vi "listbox_redrow.vi"() -> ()   [LabVIEW 2021]
panel:
  in  "Red Rows Index":i32[](array[numeric])=[1, 3, 7]
  out "Multicolumn Listbox":i32[](listbox)
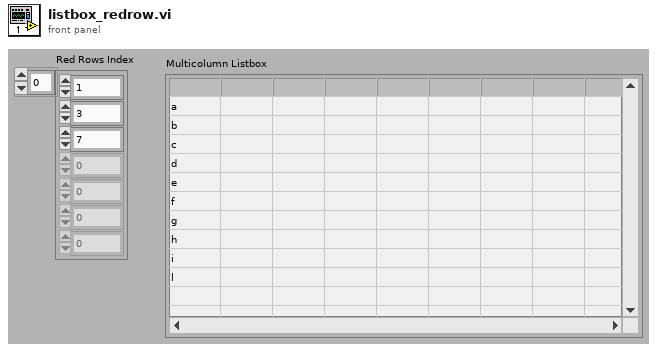
[diagram p1: front panel]
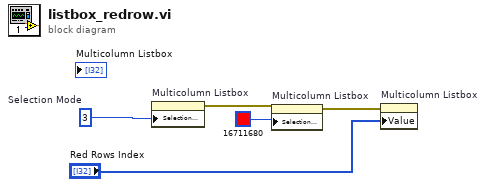
[diagram p0: block diagram]
diagram:
  w3 = 3  # Selection Mode
  n1 = property on="Multicolumn Listbox" class="MCListbox (strict)"("Selection Mode"=w3) -> (error out=w2:errorcluster)  [unwired: 2 in, 1 out]
  n2 = property on="Multicolumn Listbox" class="MCListbox (strict)"(error in=w2, "Selection Color"=u32 16711680) -> (error out=w1:errorcluster)  [unwired: 1 in, 1 out]
  n3 = property on="Multicolumn Listbox" class="MCListbox (strict)"(error in=w1, "Value"="Red Rows Index") -> ()  [unwired: 1 in, 2 out]
